vi "Queue.vi"(0 "Operation":T1, 5 "Enqueue":dbl, 7 "Size":i32, 11 "Error in":errorcluster) -> (3 "Underflow":bool, 4 "Overflow":bool, 6 "Dequeue":dbl[](array[numeric]), 8 "Queue":dbl[](array[numeric]), 10 "Sum":dbl, 15 "Error out":errorcluster)   [LabVIEW 2020]
doc: "This system does a function of storing data in the form of FIFO getting data in and out"
uses:
  Typedefs/Operations.ctl
panel:
  # "Queue"
  # "Output queue"
  # "Enter size"
  # "Dequeue"
  # "Enter element"
  # "Sum of queue"
  # "Select operation"
  # "True if overflow"
  # "True if underflow"
  # "INPUT"
  # "OUTPUT"
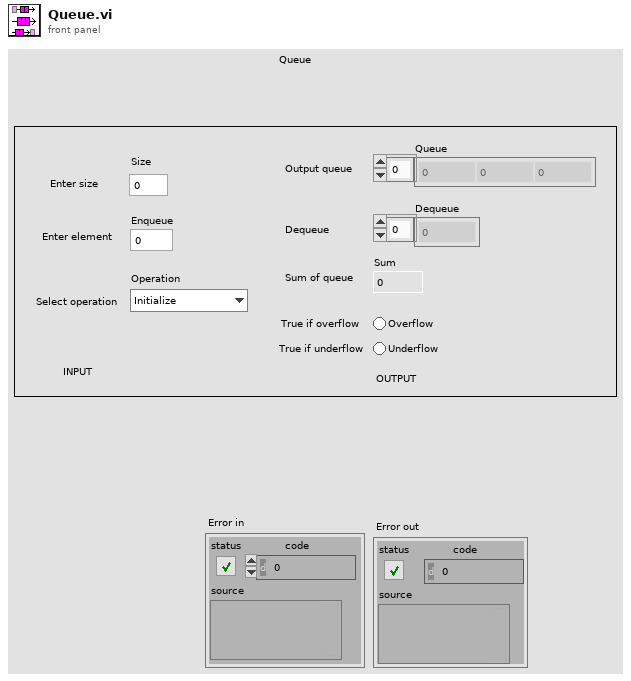
[diagram p1: front panel]
types:
  T1 = typedef "Operations.ctl" = enum16{"Initialize", "Enqueue", "Dequeue", "Sum"}
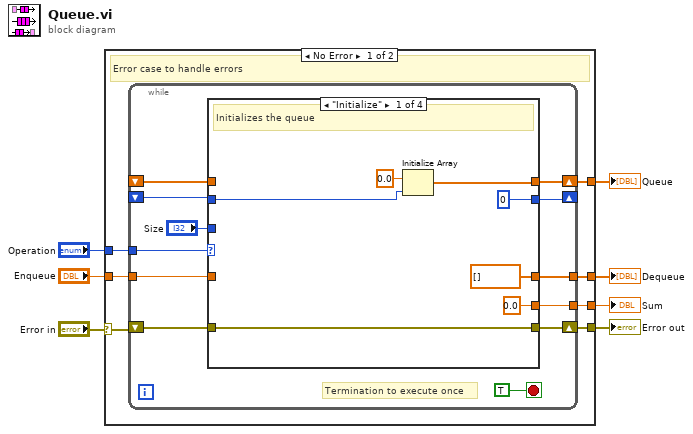
[diagram p0: block diagram]
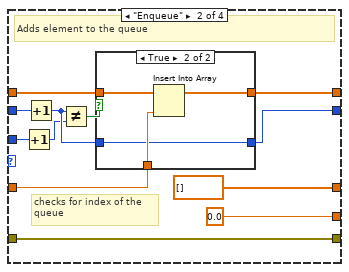
[diagram p2: hidden frame]
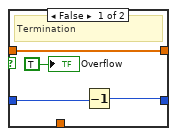
[diagram p3: hidden frame]
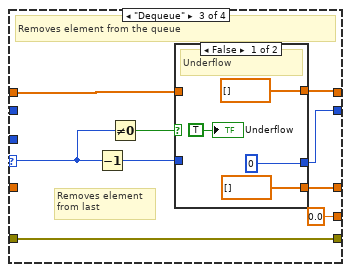
[diagram p4: hidden frame]
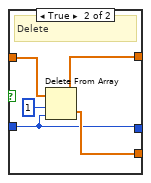
[diagram p5: hidden frame]
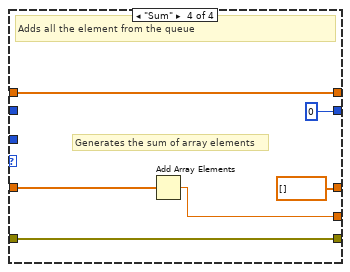
[diagram p6: hidden frame]
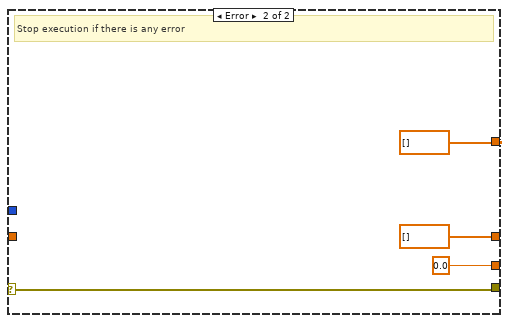
[diagram p7: hidden frame]
diagram:
  n1 = case shown="No Error" "Error in" {
    selector: "Error in" -> [w14 w80]
    tunnel: [w13 w80] -> w6
    tunnel: "Operation" -> [w12 _]
    tunnel: [w11 dbl[] []] -> w4
    tunnel: [w10 dbl[] []] -> w2
    tunnel: [w9 0.0 ("Enqueue")] -> w3
    tunnel: "Enqueue" -> [w8 _]
    frame No Error {
      # "Error case to handle errors"
      n2 = while {
        shift-right: [w24] -> w13
        shift-left: w14 -> [w25]
        shift-right: [w23] -> w10
        shift-left: _ -> [w21]
        tunnel: w12 -> [w22]
        tunnel: w8 -> [w20]
        tunnel: [w19] -> w11
        tunnel: [w18] -> w9
        shift-right: [w17] -> _
        shift-left: _ -> [w16]
        stop <- TRUE stop-if-true
        # "Termination to execute once"
        n3 = case shown="\"Initialize\"" w22 {
          tunnel: w25 -> [w33 w45 w62 w76]
          tunnel: [w33 w45 w62 w76] -> w24
          tunnel: [w32 w44 w58 w72] -> w23
          tunnel: w21 -> [_ w43 w60 w72]
          tunnel: w20 -> [_ w42 _ _]
          tunnel: [dbl[] [] dbl[] [] w61 dbl[] []] -> w19
          tunnel: w16 -> [w31 w39 w55 _]
          tunnel: [0.0 ("Enqueue") 0.0 ("Enqueue") 0.0 ("Enqueue") w75] -> w18
          tunnel: [0 w36 w54 0] -> w17
          tunnel: "Size" -> [_ w35 _ _]
          frame "Initialize" {
            # "Initializes the queue"
            n4 = Initialize Array(0.0 ("element"), w31) -> (w32:dbl[])
          }
          frame "Enqueue" {
            # "checks for index of the \nqueue"
            # "Adds element to the queue"
            n5 = Increment(x=w35) -> (x+1=w34:i32)
            n6 = Increment(x=w39) -> (x+1=w37:i32)
            n7 = Not Equal?(x=w37, y=w34) -> (x != y?=w38:bool)
            n8 = case shown="True" w38 {
              tunnel: [w49 w53] -> w44
              tunnel: w43 -> [w49 w52]
              tunnel: w42 -> [_ w51]
              tunnel: [w47 w50] -> w36
              tunnel: w37 -> [w48 w50]
              frame False {
                # "Termination"
                n9 = Decrement(x=w48) -> (x-1=w47:i32)
                "Overflow" <- TRUE ("Boolean")
              }
              frame True {
                n10 = Insert Into Array(array=w52, new element=w51) -> (w53:dbl[])  [unwired: 1 in]
              }
            }
          }
          frame "Dequeue" {
            # "Removes element \nfrom last"
            # "Removes element from the queue"
            n11 = Decrement(x=w55) -> (x-1=w57:i32)
            n12 = Not Equal To 0?(x=w55) -> (x != 0?=w56:bool)
            n13 = case shown="False" w56 {
              tunnel: [dbl[] [] w71] -> w61
              tunnel: w60 -> [_ w70]
              tunnel: [dbl[] [] w68] -> w58
              tunnel: w57 -> [_ w67]
              tunnel: [0 w67] -> w54
              frame False {
                # "Underflow"
                "Underflow" <- TRUE ("Boolean 2")
              }
              frame True {
                # "Delete"
                n14 = Delete From Array(array=w70, length=1, index=w67) -> (deleted portion=w71:dbl[], array with subset deleted=w68:dbl[])
              }
            }
          }
          frame "Sum" {
            # "Generates the sum of array elements"
            # "Adds all the element from the queue"
            n15 = Add Array Elements(numeric array=w72) -> (sum=w75:dbl)
          }
        }
      }
    }
    frame Error {
      # "Stop execution if there is any error"
    }
  }
  "Error out" <- w6
  "Dequeue" <- w4
  "Sum" <- w3
  "Queue" <- w2
